vi "FMTone-Compute Max Level.vi"(0 "FM":T3, 9 "Level":T1, 11 "error in (no error)":errorcluster, 12 "Fs (Hz)":dbl) -> (6 "Max Level":dbl, 10 "Level out":T1, 15 "error out":errorcluster)   [LabVIEW 2020]
uses:
  XControls/Waveform XControls/FM Tone/FM.Properties.ctl
  XControls/Level (G3)/Level Data.ctl
  XControls/Level (G3)/Level Units (G3).ctl
  Utility VIs/Math VIs/Linear to dB (scalar).vi
  PXI DAQ VIs/DAQ Engine VIs/PXI Globals.vi
  XControls/Level (G3)/Level (G3).xctl
  XControls/Waveform XControls/FM Tone/FM Tone.xctl
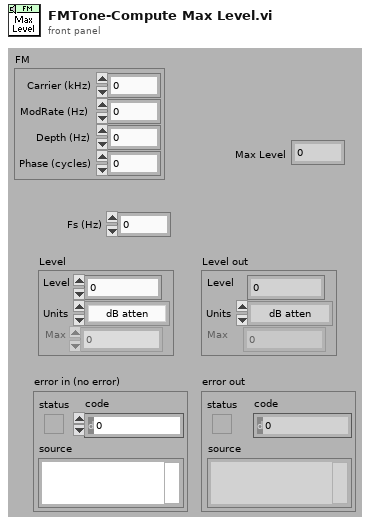
[diagram p1: front panel]
types:
  T1 = typedef "Level (G3).xctl/Level Data.ctl" = cluster{"Level":dbl, "Units":T2, "Max":dbl, "Data":cluster{"Multiplier":dbl, "Cal File":path, "Cal":cluster{"Freq (Hz)":dbl[], "Mag (dB SPL)":dbl[], "Phase (deg)":dbl[]}, "audiogram":path}}
  T2 = typedef "Level (G3).xctl/Level Units (G3).ctl" = enum16{"dB atten", "dB SPL", "dB re 1 Vrms", "dB V/Hz½", "mW", "dB HL", "Volts", "dB mW"}
  T3 = typedef "FM Tone.xctl/FM.Properties.ctl" = cluster{"Carrier (kHz)":dbl, "ModRate (Hz)":dbl, "Depth (Hz)":dbl, "Phase (cycles)":dbl}
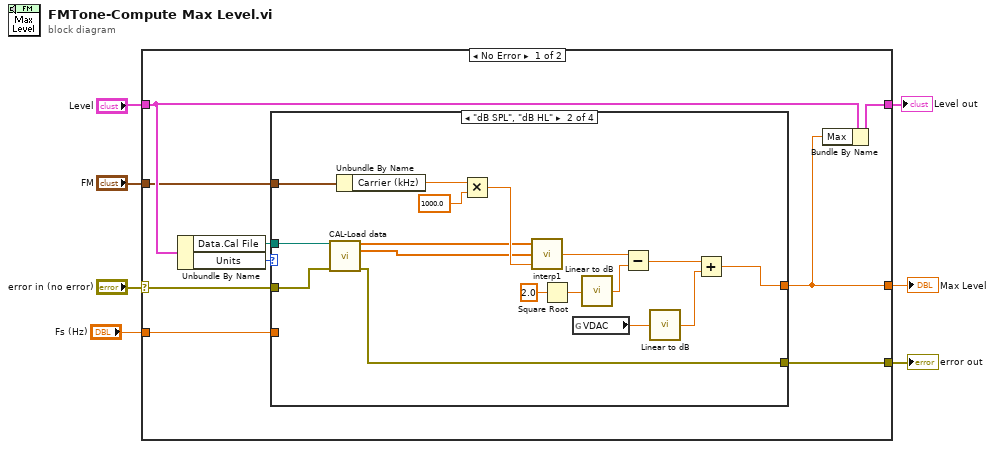
[diagram p0: block diagram]
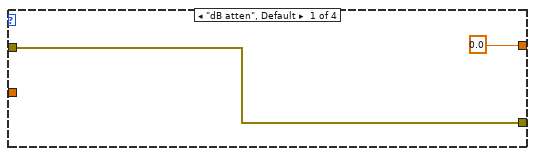
[diagram p2: hidden frame]
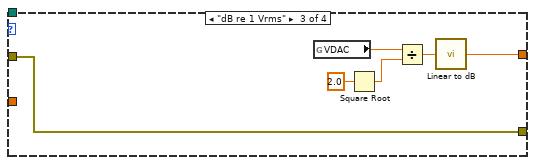
[diagram p3: hidden frame]
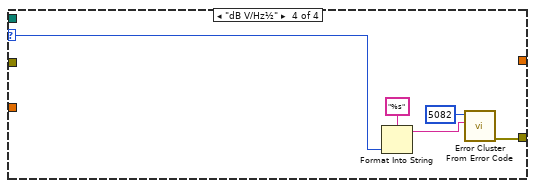
[diagram p4: hidden frame]
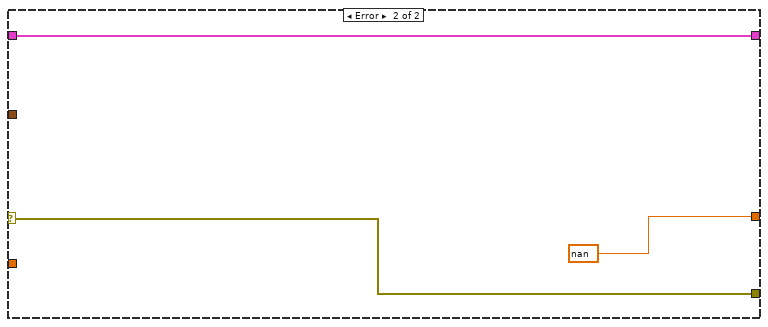
[diagram p5: hidden frame]
diagram:
  n1 = case shown="No Error" "error in (no error)" {
    selector: "error in (no error)" -> [w16 w49]
    tunnel: "Level" -> [w14 w47]
    tunnel: "FM" -> [w9 _]
    tunnel: [w15 w49] -> w6
    tunnel: [w13 nan ("Reference Level")] -> w3
    tunnel: [w12 w47] -> w2
    tunnel: "Fs (Hz)" -> [w8 _]
    frame No Error {
      n2 = Unbundle By Name(w14) -> ("Data.Cal File"=w11:path, "Units"=w10:T2)
      n3 = case shown="\"dB SPL\", \"dB HL\"" w10 {
        selector: w10 -> [_ _ _ w42]
        tunnel: w16 -> [w17 w35 w41 _]
        tunnel: w9 -> [_ w33 _ _]
        tunnel: [0.0 ("Reference Level") w34 w36 _] -> w13
        tunnel: [w17 w32 w41 w43] -> w15
        tunnel: w11 -> [_ w31 _ _]
        tunnel: w8 -> [_ _ _ _]
        frame "dB atten", Default {
        }
        frame "dB SPL", "dB HL" {
          n4 = call "CAL-Load data.vi"("user path"=w31, "error in (no error)"=w35) -> ("Frequency (Hz)"=w20:dbl[], "Mag"=w19:dbl[], "error out"=w32:errorcluster)  [unwired: 6 in, 5 out]
          n5 = Unbundle By Name(w33) -> ("Carrier (kHz)"=w28:dbl)
          n6 = Multiply(x=w28, y=1000.0) -> (x*y=w26:dbl)
          n7 = call "interp1.vi"("X"=w20, "Y"=w19, "U"=w26) -> ("V"=w24:dbl)  [unwired: 2 in]
          n8 = Square Root(x=2.0 ("y")) -> (sqrt(x)=w23:dbl)
          n9 = global read "PXI Globals.vi" "VDAC"() -> (w30:dbl)
          n10 = call-poly "Linear to dB.vi"("Linear"=w23) -> ("dB"=w22:dbl)
          n11 = Subtract(x=w24, y=w22) -> (x-y=w21:dbl)
          n12 = call-poly "Linear to dB.vi"("Linear"=w30) -> ("dB"=w29:dbl)
          n13 = Add(x=w21, y=w29) -> (x+y=w34:dbl)
        }
        frame "dB re 1 Vrms" {
          n14 = global read "PXI Globals.vi" "VDAC"() -> (w38:dbl)
          n15 = Square Root(x=2.0 ("y")) -> (sqrt(x)=w39:dbl)
          n16 = Divide(x=w38, y=w39) -> (x/y=w37:dbl)
          n17 = call-poly "Linear to dB.vi"("Linear"=w37) -> ("dB"=w36:dbl)
        }
        frame "dB V/Hz½" {
          n18 = Format Into String(format string="%s", w42) -> (resulting string=w45:string)  [unwired: 2 in, 1 out]
          n19 = call <vilib>:"Error Cluster From Error Code.vi"("error message (\"\")"=w45, "error code (0)"=5082) -> ("error out"=w43:errorcluster)  [unwired: 7 in]
        }
      }
      n20 = Bundle By Name(cluster=w14, "Max"=w13) -> (w12:T1)
    }
    frame Error {
    }
  }
  "error out" <- w6
  "Max Level" <- w3
  "Level out" <- w2
